vi "Configure Measurement Edge.vi"   [LabVIEW 2023, in "Keysight-DSQx3014T.lvlib"]
doc: "Configures the measurement edge."
uses:
  Keysight-DSQx3014T.lvlib
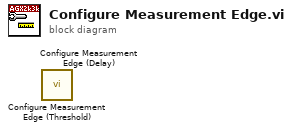
[diagram p0: block diagram]
diagram:
  n1 = call "Configure Measurement Edge (Threshold).vi"() -> ()  [unwired: 10 in, 2 out]
  n2 = call "Configure Measurement Edge (Delay).vi"() -> ()  [unwired: 10 in, 2 out]
